vi "Scan_setup.vi"(0 "X axis":T3, 1 "Y axis":T3, 4 "Z axis":T3, 5 "Initial sample rate (Hz)":dbl, 7 "error in (no error)":errorcluster, 11 "Scan mode":T1(ring)=enum."Single Direction (Uniform)", 12 "Sample clock source":tag, 13 "Lissajous Cluster":cluster{"a":dbl, "b":dbl, "delta":dbl}={"a"=1.0, "b"=2.0, "delta"=0.0} {"delta" format="%_3g"; "b" format="%0.2p"; "a" format="%_3g"}, 14 "Home the stage after scan?":bool, 15 "asymmetry":dbl=0.9, 16 "Scan dimension":T2(ring), 17 "Soften":bool, 19 "Soften points":i32=3) -> (20 "task out":refnum<k21>, 21 "Waveform Graph":dbl[][](graph), 24 "Samples per channel":i32, 25 "Actual sample rate (Hz)":dbl, 27 "error out":errorcluster)   [LabVIEW 2014]
uses:
  <vilib>/DAQmx/create/channels.llb/DAQmx Create Channel (AO-Voltage-Basic).vi
  <vilib>/DAQmx/configure/timing.llb/DAQmx Timing (Sample Clock).vi
  <vilib>/DAQmx/write.llb/DAQmx Write (Analog 2D DBL NChan NSamp).vi
  <resource>/objmgr/daqmx.rc
panel:
  out "Sample rate (Hz)":dbl
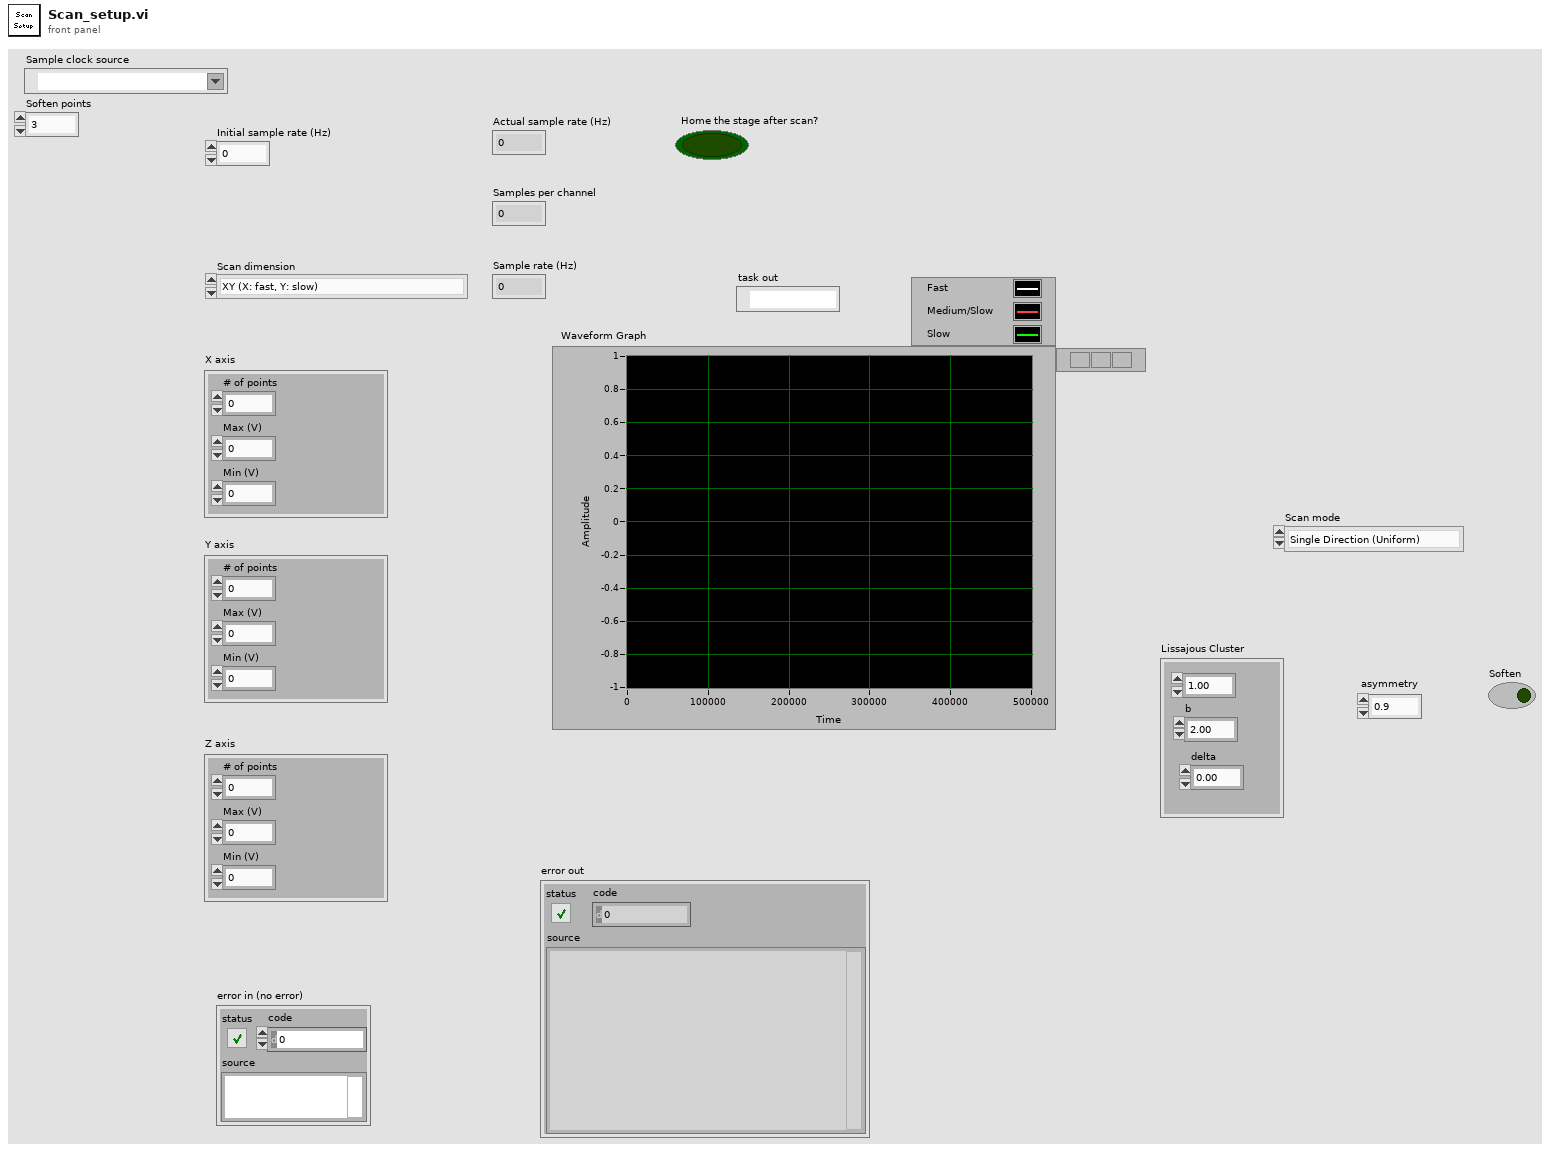
[diagram p1: front panel]
types:
  T1 = enum16{"Lissajous", "Adjustable sawtooth", "Single Direction (Uniform)", "Single Direction (Fast Reset)", "Bi-Directional"}
  T2 = enum8{"XY (X: fast, Y: slow)", "XYZ (X: fast, Y: medium, Z: slow)"}
  T3 = cluster{"# of points":u16, "Max (V)":dbl, "Min (V)":dbl}
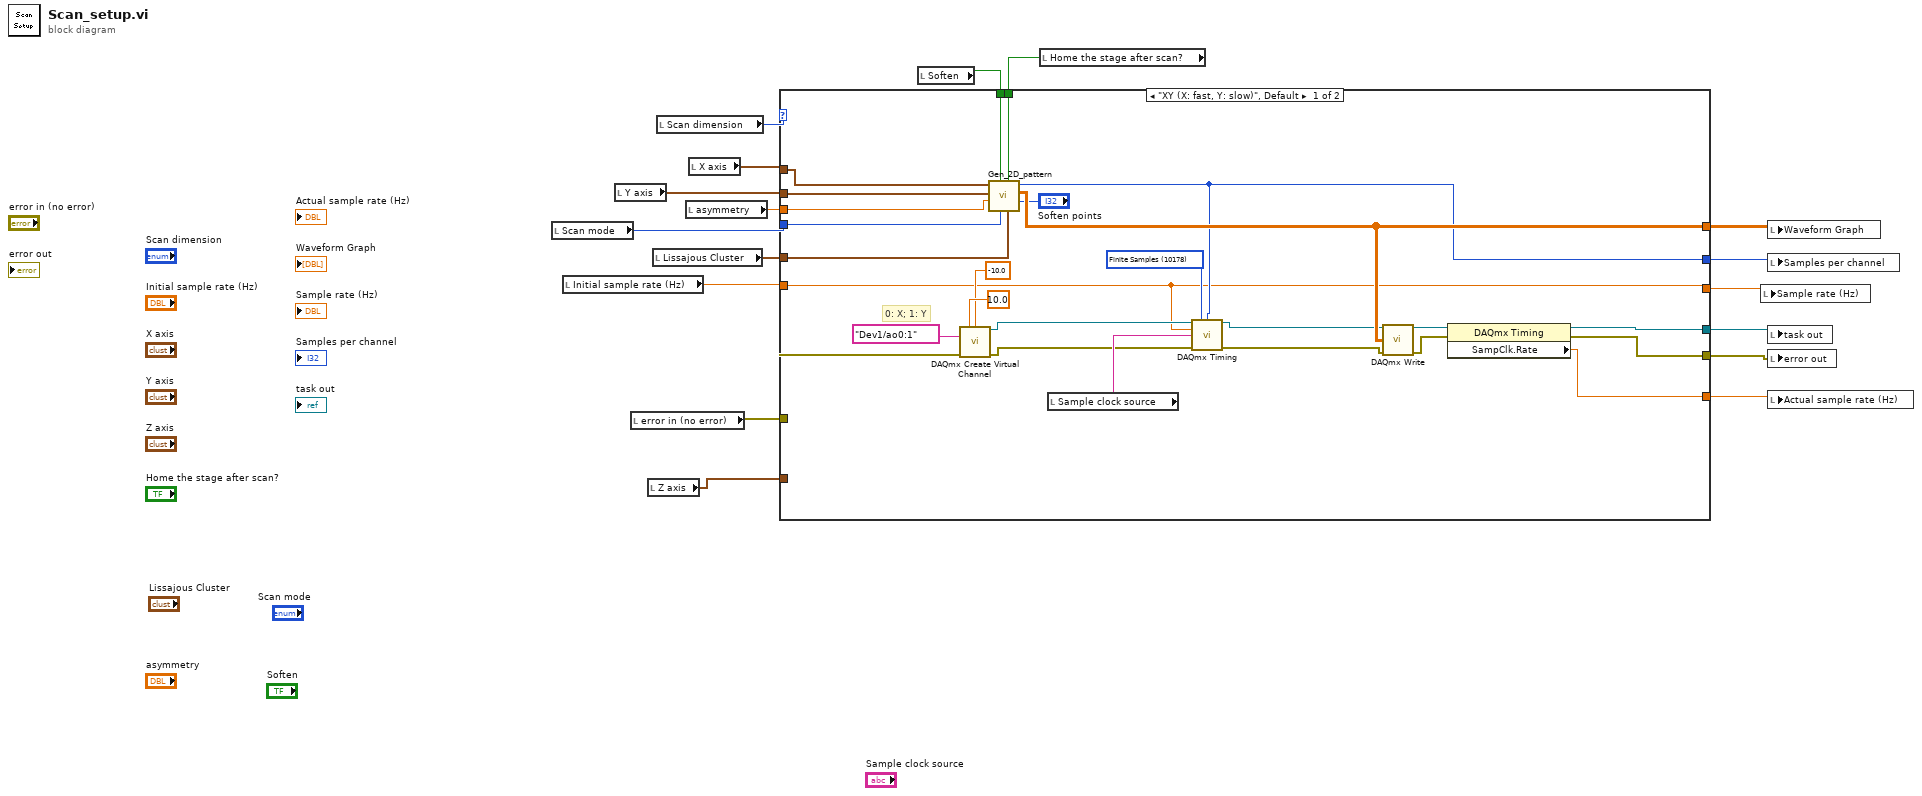
[diagram p0: block diagram]
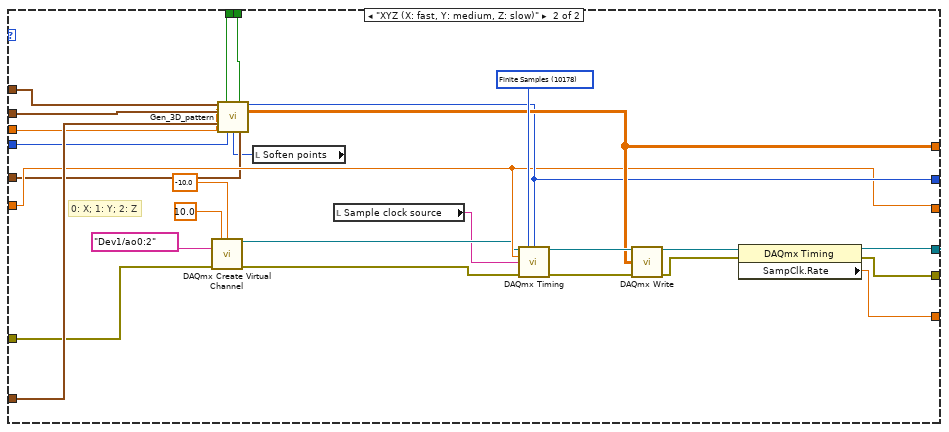
[diagram p2: hidden frame]
diagram:
  n1 = local read "Scan mode"() -> (w3:T1)
  n2 = local read "Initial sample rate (Hz)"() -> (w7:dbl)
  n3 = local read "Y axis"() -> (w15:T3)
  n4 = local read "error in (no error)"() -> (w14:errorcluster)
  n5 = local read "Z axis"() -> (w17:T3)
  n6 = local read "Lissajous Cluster"() -> (w2:cluster{"a":dbl, "b":dbl, "delta":dbl})
  n7 = local read "Scan dimension"() -> (w16:T2)
  n8 = local read "asymmetry"() -> (w1:dbl)
  n9 = local read "X axis"() -> (w5:T3)
  n10 = local read "Soften"() -> (w4:bool)
  n11 = local read "Home the stage after scan?"() -> (w6:bool)
  n12 = case shown="\"XY (X: fast, Y: slow)\", Default" w16 {
    tunnel: w7 -> [w24 w54]
    tunnel: w17 -> [_ w60]
    tunnel: w5 -> [w36 w62]
    tunnel: w15 -> [w35 w61]
    tunnel: w3 -> [w22 w48]
    tunnel: w14 -> [w37 w52]
    tunnel: [w33 w57] -> w13
    tunnel: [w34 w59] -> w12
    tunnel: [w31 w58] -> w11
    tunnel: [w32 w56] -> w10
    tunnel: [w30 w55] -> w9
    tunnel: [w24 w54] -> w8
    tunnel: w6 -> [w23 w53]
    tunnel: w4 -> [w21 w46]
    tunnel: w2 -> [w20 w45]
    tunnel: w1 -> [w19 w47]
    frame "XY (X: fast, Y: slow)", Default {
      w40 = 10178 items=["Finite Samples"=10178, "Continuous Samples"=10123, "Hardware Timed Single Point"=12522] ("sample mode")
      # "0: X; 1: Y"
      n13 = call-poly <vilib>:"DAQmx Create Virtual Channel.vi"("maximum value"=10.0, "minimum value"=-10.0, "physical channels"=tag "Dev1/ao0:1", "error in"=w37) -> ("task out"=w28:refnum<k21>, "error out"=w27:errorcluster)  [unwired: 10 in]
      n14 = call "Gen_2D_pattern.vi"("Soften points"="Soften points", "Lissajous Cluster"=w20, "Home the stage after scan?"=w23, "Scan mode"=w22, "Soften"=w21, "asymmetry"=w19, "Slow axis"=w35, "Fast axis"=w36) -> ("Waveform Graph"=w31:dbl[][], "Samples per channel"=w30:i32)  [unwired: 1 in, 1 out]
      n15 = local read "Sample clock source"() -> (w29:tag)
      n16 = call-poly <vilib>:"DAQmx Timing.vi"("task/channels in"=w28, "sample mode"=w40, "samples per channel"=w30, "rate"=w24, "source"=w29, "error in"=w27) -> ("task out"=w26:refnum<k21>, "error out"=w25:errorcluster)  [unwired: 8 in]
      n17 = call-poly <vilib>:"DAQmx Write.vi"("task/channels in"=w26, "data"=w31, "error in"=w25) -> ("task out"=w39:refnum<k21>, "error out"=w38:errorcluster)  [unwired: 10 in, 1 out]
      n18 = property class="DAQmx Timing"(reference=w39, error in=w38) -> (reference out=w32:refnum<k21>, error out=w33:errorcluster, "SampClk.Rate"=w34:dbl)
    }
    frame "XYZ (X: fast, Y: medium, Z: slow)" {
      w66 = 10178 items=["Finite Samples"=10178, "Continuous Samples"=10123, "Hardware Timed Single Point"=12522] ("sample mode")
      # "0: X; 1: Y; 2: Z"
      n19 = call-poly <vilib>:"DAQmx Create Virtual Channel.vi"("maximum value"=10.0, "minimum value"=-10.0, "physical channels"=tag "Dev1/ao0:2", "error in"=w52) -> ("task out"=w51:refnum<k21>, "error out"=w50:errorcluster)  [unwired: 10 in]
      n20 = local read "Soften points"() -> (w44:i32)
      n21 = call "Gen_3D_pattern.vi"("X: fast axis"=w62, "asymmetry"=w47, "Home the stage after scan?"=w53, "Y: points"=w61, "Z: points"=w60, "Soften"=w46, "Scan mode"=w48, "Soften points"=w44, "Lissajous Cluster"=w45) -> ("Samples per channel"=w55:i32, "Scan pattern"=w58:dbl[][])  [unwired: 4 in, 1 out]
      n22 = local read "Sample clock source"() -> (w49:tag)
      n23 = call-poly <vilib>:"DAQmx Timing.vi"("task/channels in"=w51, "sample mode"=w66, "samples per channel"=w55, "rate"=w54, "source"=w49, "error in"=w50) -> ("task out"=w67:refnum<k21>, "error out"=w68:errorcluster)  [unwired: 8 in]
      n24 = call-poly <vilib>:"DAQmx Write.vi"("task/channels in"=w67, "data"=w58, "error in"=w68) -> ("task out"=w69:refnum<k21>, "error out"=w70:errorcluster)  [unwired: 10 in, 1 out]
      n25 = property class="DAQmx Timing"(reference=w69, error in=w70) -> (reference out=w56:refnum<k21>, error out=w57:errorcluster, "SampClk.Rate"=w59:dbl)
    }
  }
  n26 = local write "Sample rate (Hz)"(w8) -> ()
  n27 = local write "Waveform Graph"(w11) -> ()
  n28 = local write "Samples per channel"(w9) -> ()
  n29 = local write "task out"(w10) -> ()
  n30 = local write "error out"(w13) -> ()
  n31 = local write "Actual sample rate (Hz)"(w12) -> ()
